vi "events.get.vi"(11 "librarian_sm in":refnum<class "librarian.lvclass">) -> (2 "events":T1, 3 "librarian_sm out":refnum<class "librarian.lvclass">)   [LabVIEW 2020, in "librarian.lvclass"]
uses:
  librarian.lvclass
  librarian.lvclass/librarian.ctl
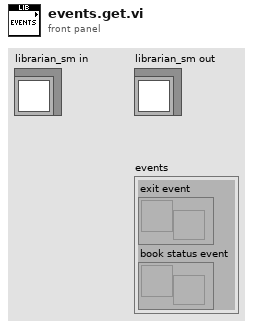
[diagram p1: front panel]
types:
  T1 = cluster{"exit event":refnum<user-event>, "book status event":refnum<user-event>}
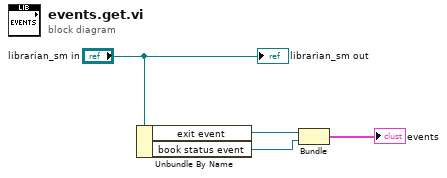
[diagram p0: block diagram]
diagram:
  n1 = Unbundle By Name("librarian_sm in") -> ("exit event"=w3:refnum<user-event>, "book status event"=w2:refnum<user-event>)
  n2 = Bundle("exit event"=w3, "book status event"=w2) -> (→"events":T1)  [unwired: 1 in]
  "librarian_sm out" <- "librarian_sm in"
